vi "PH_OceanOpticsSpectrometer.Init Spectrometer.vi"(0 "i ref in":refnum<vi>, 5 "error in":errorcluster) -> (14 "i ref out":refnum<vi>, 19 "error out":errorcluster)   [LabVIEW 2014, in "PH_OceanOpticsSpectrometer.lvlib"]
doc: "Within this VI the hardware is inizialized."
uses:
  PH_OceanOpticsSpectrometer.lvlib
  PH_StatusHandler/PH_StatusHandler.Status.ctl
  CSCore/BaseProcess/BaseProcess.lvlib
  non_GPL/instr.lib/Ocean Optics 2000 4000/Ocean Optics 2000 4000 - Driver np.lvlib
  PH_StatusHandler/PH_StatusHandler.lvlib
  PH_Common/PH_Common.lvlib
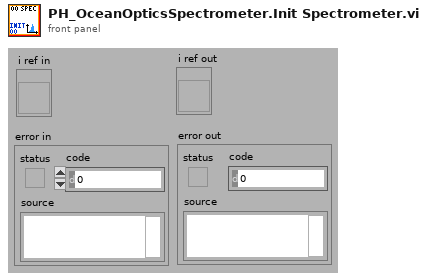
[diagram p1: front panel]
types:
  T1 = typedef "PH_OceanOpticsSpectrometer.lvlib/PH_OceanOpticsSpectrometer.i attribute.ctl" = cluster{"GUI Refs":cluster{"Delete":refnum<vi>, "Spectrum":refnum<vi>, "Display Width":refnum<vi>, "Display Center":refnum<vi>, "Save":refnum<vi>, "Integration time":refnum<vi>, "center wavelength":refnum<vi>, "width":refnum<vi>, "Wanted Trigger Mode":refnum<vi>, "Current Trigger Mode":refnum<vi>, "Trigger Info":refnum<vi>, "Model":refnum<vi>, "Driver":refnum<vi>, "Firmware":refnum<vi>}, "Display":cluster{"Width":dbl, "Center":dbl}, "VISA resource name":refnum<visa-resource-name>, "Integration time [ms]":cluster{"Current Value":u16, "Wanted Value":u16}, "Trigger":cluster{"Current value":T2, "Wanted value":T2}, "Default VISA Timeout":u32, "Last Data":cluster{"Wavelength Bins":dbl[], "Spectrum by Pixels":dbl[]}}
  T2 = typedef "PH_OceanOpticsSpectrometer.lvlib/PH_OceanOpticsSpectrometer.Trigger.ctl" = enum32{"External", "Normal"}
  T3 = typedef "PH_StatusHandler.lvlib/PH_StatusHandler.Status.ctl" = i16
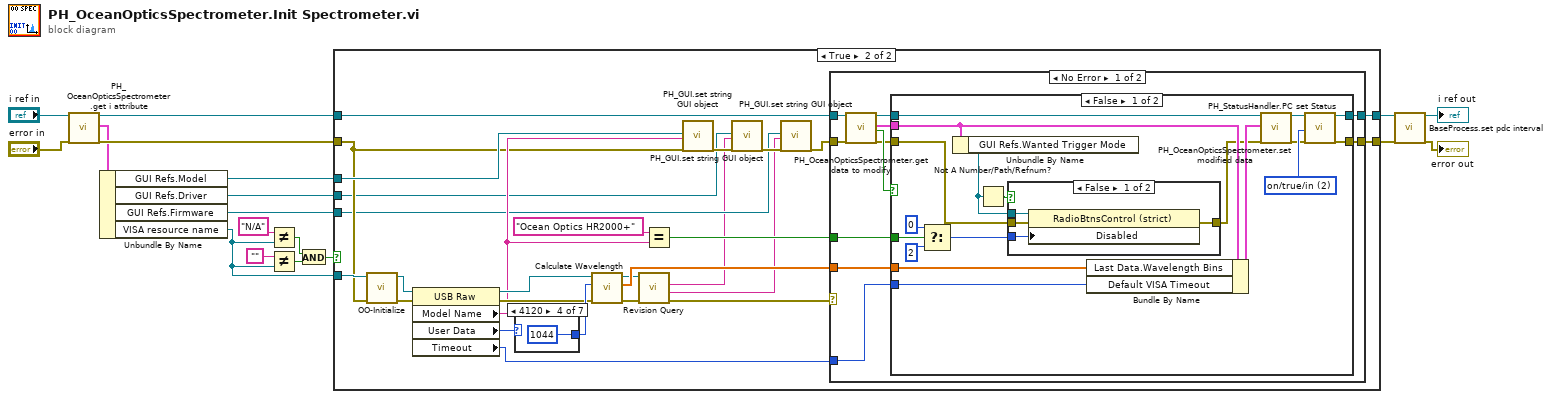
[diagram p0: block diagram]
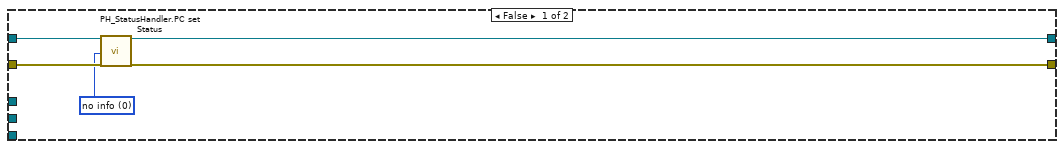
[diagram p2: hidden frame]
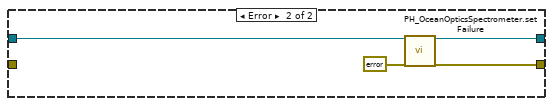
[diagram p5: hidden frame]
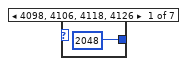
[diagram p6: hidden frame]
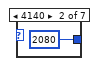
[diagram p7: hidden frame]
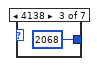
[diagram p8: hidden frame]
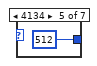
[diagram p9: hidden frame]
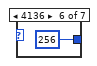
[diagram p10: hidden frame]
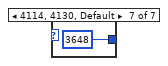
[diagram p11: hidden frame]
diagram:
  n1 = call "PH_OceanOpticsSpectrometer.get i attribute.vi"("i ref in"="i ref in", "error in (no error)"="error in") -> ("i ref out"=w5:refnum<vi>, "i attribute"=w13:T1, "error out"=w17:errorcluster)  [unwired: 15 in]
  n2 = Unbundle By Name(w13) -> ("GUI Refs.Model"=w3:refnum<vi>, "GUI Refs.Driver"=w2:refnum<vi>, "GUI Refs.Firmware"=w1:refnum<vi>, "VISA resource name"=w7:refnum<visa-resource-name>)
  n3 = Not Equal?(x="N/A", y=w7) -> (x != y?=w10:bool)
  n4 = Not Equal?(x="", y=w7) -> (x != y?=w9:bool)
  n5 = And(x=w10, y=w9) -> (x .and. y?=w8:bool)
  n6 = case shown="True" w8 {
    tunnel: w17 -> [w22 w34]
    tunnel: [w19 w50] -> w6
    tunnel: w7 -> [_ w49]
    tunnel: w5 -> [w23 w48]
    tunnel: [w20 w47] -> w4
    tunnel: w3 -> [_ w36]
    tunnel: w2 -> [_ w28]
    tunnel: w1 -> [_ w27]
    frame False {
      w21 = T3 0 items=["no info", "off/false/out", "on/true/in", "Failure", "Alarm", "Status 1", "Status 2", "Status 3"] ("Device Status")
      n7 = call "PH_StatusHandler.PC set Status.vi"("i ref in"=w23, "Status"=w21, "error in (no error)"=w22) -> ("i ref out"=w20:refnum<vi>, "error out"=w19:errorcluster)  [unwired: 15 in]
    }
    frame True {
      n8 = call "OO-Initialize.vi"("error in (no error)"=w34, "VISA resource name"=w49) -> ("error out"=w40:errorcluster, "VISA resource name out"=w41:refnum<visa-resource-name>)  [unwired: 8 in]
      n9 = property class="USB Raw"(reference=w41, error in=w40) -> (reference out=w39:refnum<visa-resource-name>, error out=w38:errorcluster, "Model Name"=w35:string, "User Data"=w42:u32, "Timeout"=w37:u32)
      n10 = case shown="4120" w42 {
        tunnel: [2048 ("Number of Pixels (3840)") 2080 ("Number of Pixels (3840)") 2068 ("Number of Pixels (3840)") 1044 ("Number of Pixels (3840)") 512 ("Number of Pixels (3840)") 256 ("Number of Pixels (3840)") 3648 ("Number of Pixels (3840)")] -> w46
        frame 4098, 4106, 4118, 4126 {
        }
        frame 4140 {
        }
        frame 4138 {
        }
        frame 4120 {
        }
        frame 4134 {
        }
        frame 4136 {
        }
        frame 4114, 4130, Default {
        }
      }
      n11 = call "Calculate Wavelength.vi"("error in (no error)"=w38, "Number of Pixels (3648)"=w46, "VISA resource name"=w39) -> ("error out"=w32:errorcluster, "Wavelength (nm)"=w44:dbl[], "VISA resource name out"=w33:refnum<visa-resource-name>)  [unwired: 6 in]
      n12 = call "Revision Query.vi"("error in (no error)"=w32, "VISA resource name"=w33) -> ("error out"=w26:errorcluster, "Instrument Firmware Revision"=w24:string, "Instrument Driver Revision"=w25:string)  [unwired: 6 in, 1 out]
      n13 = Equal?(x="Ocean Optics HR2000+", y=w35) -> (x = y?=w43:bool)
      n14 = call "PH_GUI.set string GUI object.vi"("GUI object Ref"=w36, "Text"=w35, "error in"=w34) -> ("error out"=w31:errorcluster)  [unwired: 16 in]
      n15 = call "PH_GUI.set string GUI object.vi"("GUI object Ref"=w28, "Text"=w25, "error in"=w31) -> ("error out"=w30:errorcluster)  [unwired: 16 in]
      n16 = call "PH_GUI.set string GUI object.vi"("GUI object Ref"=w27, "Text"=w24, "error in"=w30) -> ("error out"=w29:errorcluster)  [unwired: 16 in]
      n17 = case shown="No Error" w26 {
        tunnel: [w53 w87] -> w50
        tunnel: w48 -> [w61 w89]
        tunnel: [w60 w88] -> w47
        tunnel: w44 -> [w59 _]
        tunnel: w43 -> [w58 _]
        tunnel: w37 -> [w55 _]
        tunnel: w29 -> [w51 _]
        frame No Error {
          n18 = call "PH_OceanOpticsSpectrometer.get data to modify.vi"("i ref in"=w61, "error in (no error)"=w51) -> ("i ref out"=w57:refnum<vi>, "i attribute"=w56:T1, "timed out"=w54:bool, "error out"=w52:errorcluster)  [unwired: 14 in]
          n19 = case shown="False" w54 {
            tunnel: [w64 w86] -> w60
            tunnel: w59 -> [w69 _]
            tunnel: w58 -> [w75 _]
            tunnel: w57 -> [w74 w86]
            tunnel: w56 -> [w73 _]
            tunnel: w55 -> [w71 _]
            tunnel: [w62 w85] -> w53
            tunnel: w52 -> [w68 w85]
            frame False {
              w67 = T3 2 items=["no info", "off/false/out", "on/true/in", "Failure", "Alarm", "Status 1", "Status 2", "Status 3"] ("Device Status")
              n20 = Select(t=u8 0, s=w75, f=u8 2) -> (s? t:f=w79:u8)
              n21 = Unbundle By Name(w73) -> ("GUI Refs.Wanted Trigger Mode"=w70:refnum<vi>)
              n22 = Not A Number/Path/Refnum?(number/path/refnum=w70) -> (NaN/Path/Refnum?=w78:bool)
              n23 = case shown="False" w78 {
                tunnel: w68 -> [w83 w84]
                tunnel: [w82 w84] -> w66
                tunnel: w70 -> [w81 _]
                tunnel: w79 -> [w80 _]
                frame False {
                  n24 = property class="RadioBtnsControl (strict)"(reference=w81, error in=w83, "Disabled"=w80) -> (error out=w82:errorcluster)  [unwired: 1 out]
                }
                frame True {
                }
              }
              n25 = Bundle By Name(cluster=w73, "Last Data.Wavelength Bins"=w69, "Default VISA Timeout"=w71) -> (w72:T1)
              n26 = call "PH_OceanOpticsSpectrometer.set modified data.vi"("i ref in"=w74, "i attribute"=w72, "error in (no error)"=w66) -> ("i ref out"=w65:refnum<vi>, "error out"=w63:errorcluster)  [unwired: 15 in]
              n27 = call "PH_StatusHandler.PC set Status.vi"("i ref in"=w65, "Status"=w67, "error in (no error)"=w63) -> ("i ref out"=w64:refnum<vi>, "error out"=w62:errorcluster)  [unwired: 15 in]
            }
            frame True {
            }
          }
        }
        frame Error {
          n28 = call "PH_OceanOpticsSpectrometer.set Failure.vi"("i ref in"=w89, "error IO"=errorcluster {"status"=FALSE, "code"=0, "source"=""} ("error out")) -> ("i ref out"=w88:refnum<vi>, "error out"=w87:errorcluster)  [unwired: 16 in]
        }
      }
    }
  }
  n29 = call "BaseProcess.set pdc interval.vi"("i ref in"=w4, "error in (no error)"=w6) -> ("i ref out"=→"i ref out":refnum<vi>, "error out"=→"error out":errorcluster)  [unwired: 15 in, 1 out]
